vi "Set Local Variables from DB Values.vi"(6 "Local Variable Top Level":string, 8 "error in (no error)":errorcluster, 9 "Dictionary Keys":string[](array[string]), 10 "Local Variable Mapping":string[](array[string]), 11 "QPA Measurement in":refnum<class "QPA Measurement.lvclass">) -> (0 "error out":errorcluster, 3 "QPA Measurement out":refnum<class "QPA Measurement.lvclass">)   [LabVIEW 2016, in "QPA Measurement.lvlib" / "QPA Measurement.lvclass"]
uses:
  QPA Measurement.lvclass
  C:/Projects/STS/Common/Sequence Automation/Plugins/Measurement Interface.lvlibp/Measurement Interface.lvclass
  Plugins/Measurement Interface.lvlibp/Private Methods/Measurement Parameters/Read Measurement Parameters.vi
  Plugins/String Database.lvlibp/String Database.lvclass
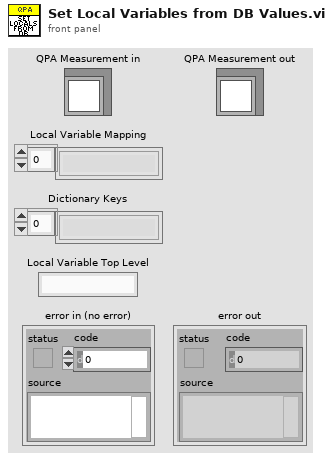
[diagram p1: front panel]
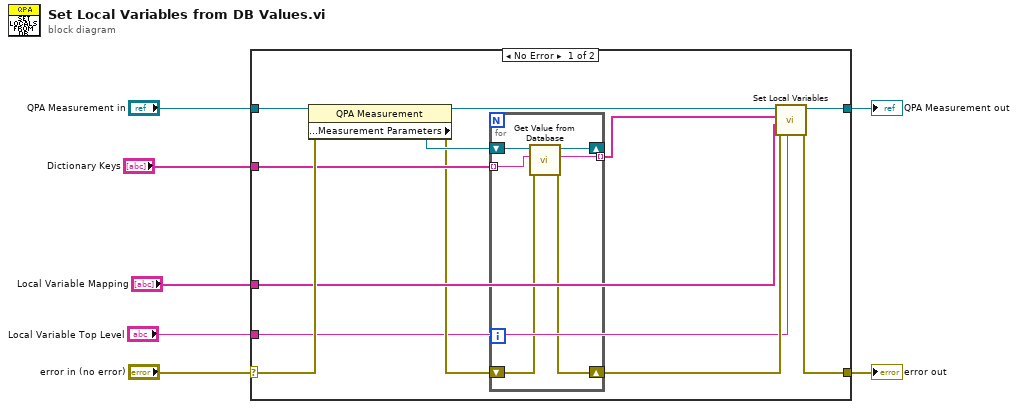
[diagram p0: block diagram]
diagram:
  n1 = case shown="No Error" "error in (no error)" {
    selector: "error in (no error)" -> [w19 w27]
    tunnel: [w18 w27] -> w6
    tunnel: [w17 w26] -> w4
    tunnel: "QPA Measurement in" -> [w16 w26]
    tunnel: "Local Variable Mapping" -> [w12 _]
    tunnel: "Dictionary Keys" -> [w11 _]
    tunnel: "Local Variable Top Level" -> [w8 _]
    frame No Error {
      n2 = property class="QPA Measurement"(reference=w16, error in=w19) -> (reference out=w15:refnum<class "QPA Measurement.lvclass">, error out=w10:errorcluster, "Protected Methods:Measurement Parameters"=w14:refnum<class "String Database.lvclass">)
      n3 = for {
        shift-right: [w24] -> _
        shift-left: w14 -> [w25]
        tunnel: [w23] -> w13 mode=indexing
        tunnel: w11 -> [w22] mode=indexing
        shift-right: [w21] -> w9
        shift-left: w10 -> [w20]
        n4 = call "Get Value from Database.vi"("error in (no error)"=w20, "Entry Name"=w22, "Message in"=w25) -> ("error out"=w21:errorcluster, "Entry Value"=w23:string, "Message out"=w24:refnum<class "String Database.lvclass">)  [unwired: 5 in, 1 out]
      }
      n5 = call "Set Local Variables.vi"("Local Variable Top Level"=w8, "error in (no error)"=w9, "Local Variable Mapping"=w12, "Values(As String)"=w13, "QPA Measurement In"=w15) -> ("error out"=w18:errorcluster, "QPA Measurement Out"=w17:refnum<class "QPA Measurement.lvclass">)  [unwired: 5 in]
    }
    frame Error {
    }
  }
  "error out" <- w6
  "QPA Measurement out" <- w4
